vi "CaseStatement2.vi"() -> ()   [LabVIEW 2014]
panel:
  in  "0=Add, 1=Subtract, 2=Mult":i32
  out "Result":dbl
  in  "B":dbl
  in  "A":dbl
  out "Multiplied":bool
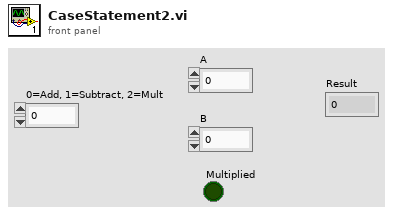
[diagram p1: front panel]
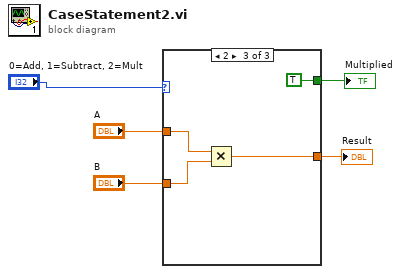
[diagram p0: block diagram]
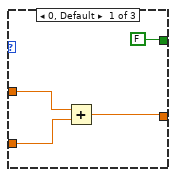
[diagram p2: hidden frame]
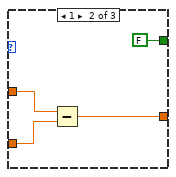
[diagram p3: hidden frame]
diagram:
  n1 = case shown="2" "0=Add, 1=Subtract, 2=Mult" {
    tunnel: "A" -> [w9 w13 w17]
    tunnel: "B" -> [w8 w12 w16]
    tunnel: [w7 w11 w15] -> w3
    tunnel: [FALSE FALSE TRUE] -> w2
    frame 0, Default {
      n2 = Add(x=w9, y=w8) -> (x+y=w7:dbl)
    }
    frame 1 {
      n3 = Subtract(x=w13, y=w12) -> (x-y=w11:dbl)
    }
    frame 2 {
      n4 = Multiply(x=w17, y=w16) -> (x*y=w15:dbl)
    }
  }
  "Multiplied" <- w2
  "Result" <- w3
